vi "Request Imaging Data.vi"(11 "Imaging data address in":u32) -> (1 "Imaging data address in indicator":u32, 3 "Imaging data address out":u32)   [LabVIEW 2015]
uses:
  OpenScan Labview code_20170126/Global_Sample per Frame.vi
  <vilib>/rvi/Memory/Memory_Emulation/niFpgaMemoryFastEmulationDramWriteAndRequestData.vi
  <vilib>/rvi/Memory/Memory_Emulation/niFpgaMemoryEmulationDramWriteAndRequestData.vi
  <vilib>/rvi/DataTransferAndStorage/Container/Common/niFpgaContainerGetUniqueNameForEmu.vi
  <vilib>/rvi/Memory/Memory_Emulation/niFpgaMemoryEmulationDramWriteAndRequestDataApplyByteEnables.vi
  <vilib>/rvi/DataTransferAndStorage/Container/XNode/niFpgaContainer.xnode
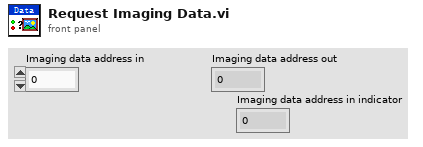
[diagram p1: front panel]
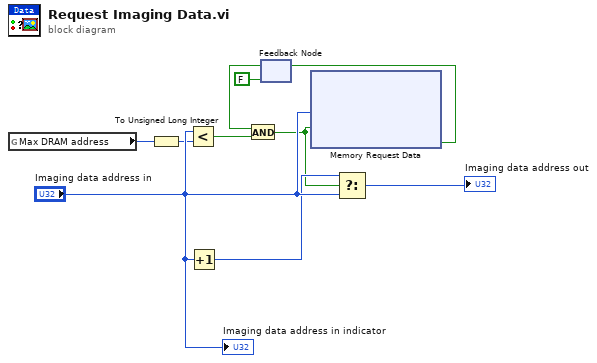
[diagram p0: block diagram]
diagram:
  n1 = global read "Global_Sample per Frame.vi" "Max DRAM address"() -> (w8:u32)
  n2 = To Unsigned Long Integer(number=w8) -> (unsigned 32bit integer=w6:u32)
  n3 = Less?(x="Imaging data address in", y=w6) -> (x < y?=w1:bool)
  n4 = Increment(x="Imaging data address in") -> (x+1=w5:u32)
  n5 = feedback #1(FALSE ("Ready for Input")) -> (w3:bool)
  n6 = And(x=w3, y=w1) -> (x .and. y?=w4:bool)
  n7 = xnode ("Memory Request Data")("Address"="Imaging data address in", "Input Valid"=w4) -> ("Ready for Input"=w2:bool)  [unwired: 1 in, 1 out]
  n8 = feedback-in #1(w2) -> ()
  n9 = Select(t=w5, s=w4, f="Imaging data address in") -> (s? t:f=→"Imaging data address out":u32)
  "Imaging data address in indicator" <- "Imaging data address in"
